vi "Draw Overlay.vi"(10 "OverlayIndex":dbl, 11 "Refnum in":T1) -> (3 "Refnum out":T1)   [LabVIEW 2016]
uses:
  <vilib>/vision/Image Controls.llb/IMAQ Image.ctl
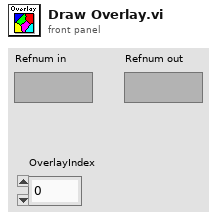
[diagram p1: front panel]
types:
  T1 = typedef "IMAQ Image.ctl" = refnum<image>
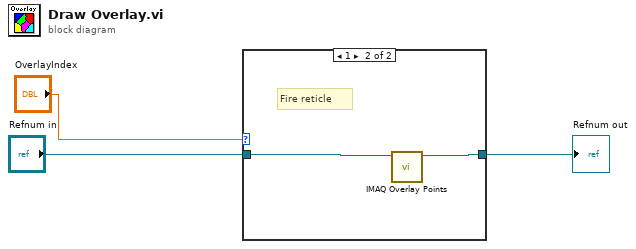
[diagram p0: block diagram]
diagram:
  n1 = case shown="1" "OverlayIndex" {
    tunnel: [w4 w6] -> w3
    tunnel: "Refnum in" -> [w4 w5]
    frame 0, Default {
      # "Draw rien"
    }
    frame 1 {
      # "Fire reticle"
      n2 = call "IMAQ Overlay Points"("Image"=w5) -> ("Image Out"=w6:T1)  [unwired: 9 in, 1 out]
    }
  }
  "Refnum out" <- w3
